vi "UAGetXMLData.vi"(8 "error in (no error)":errorcluster, 11 "String":string) -> (0 "error out":errorcluster, 3 "Server config info":T1)   [LabVIEW 2014, in "OPCUA XML.lvlib"]
uses:
  OPCUA XML.lvlib
  DEF-Server Config Data.ctl
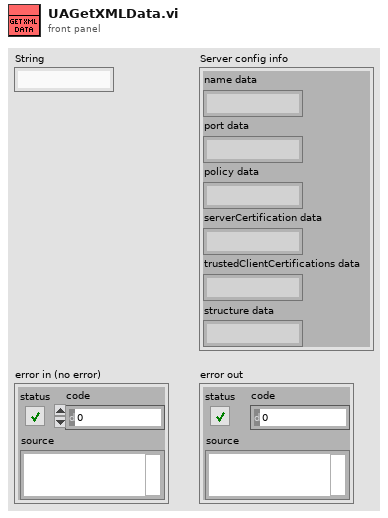
[diagram p1: front panel]
types:
  T1 = typedef "OPCUA XML.lvlib/DEF-Server Config Data.ctl" = cluster{"name data":string, "port data":string, "policy data":string, "serverCertification data":string, "trustedClientCertifications data":string, "structure data":string}
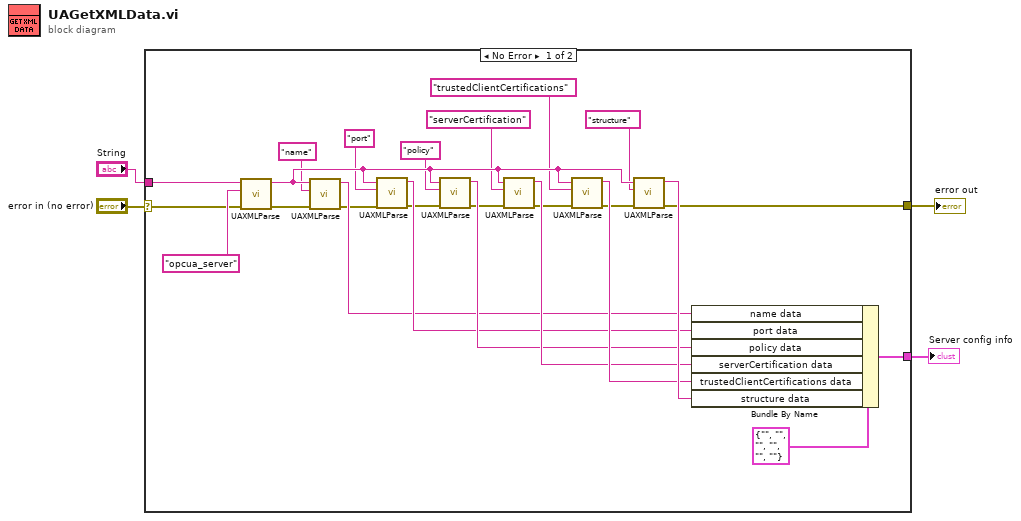
[diagram p0: block diagram]
diagram:
  n1 = case shown="No Error" "error in (no error)" {
    selector: "error in (no error)" -> [w5 w30]
    tunnel: [w28 _] -> w4
    tunnel: [w22 w30] -> w3
    tunnel: "String" -> [w6 _]
    frame No Error {
      n2 = call "UAXMLParse.vi"("error in (no error)"=w5, "label"="opcua_server", "string"=w6) -> ("error out"=w8:errorcluster, "content"=w15:string)  [unwired: 3 in, 4 out]
      n3 = call "UAXMLParse.vi"("error in (no error)"=w8, "label"="name", "string"=w15) -> ("error out"=w16:errorcluster, "content"=w23:string)  [unwired: 3 in, 4 out]
      n4 = call "UAXMLParse.vi"("error in (no error)"=w16, "label"="port", "string"=w15) -> ("error out"=w17:errorcluster, "content"=w24:string)  [unwired: 3 in, 4 out]
      n5 = call "UAXMLParse.vi"("error in (no error)"=w17, "label"="policy", "string"=w15) -> ("error out"=w18:errorcluster, "content"=w25:string)  [unwired: 3 in, 4 out]
      n6 = call "UAXMLParse.vi"("error in (no error)"=w18, "label"="serverCertification", "string"=w15) -> ("error out"=w19:errorcluster, "content"=w26:string)  [unwired: 3 in, 4 out]
      n7 = call "UAXMLParse.vi"("error in (no error)"=w19, "label"="trustedClientCertifications", "string"=w15) -> ("error out"=w20:errorcluster, "content"=w27:string)  [unwired: 3 in, 4 out]
      n8 = call "UAXMLParse.vi"("error in (no error)"=w20, "label"="structure", "string"=w15) -> ("error out"=w22:errorcluster, "content"=w29:string)  [unwired: 3 in, 4 out]
      n9 = Bundle By Name(cluster=T1 {"name data"="", "port data"="", "policy data"="", "serverCertification data"="", "trustedClientCertifications data"="", "structure data"=""} ("Server config info"), "name data"=w23, "port data"=w24, "policy data"=w25, "serverCertification data"=w26, "trustedClientCertifications data"=w27, "structure data"=w29) -> (w28:T1)
    }
    frame Error {
    }
  }
  "Server config info" <- w4
  "error out" <- w3
